vi "Vision Research Phantom Series PhCon Error Handler.vi"(0 "ErrNo":u32, 5 "Error In (no error)":errorcluster) -> (19 "Error Out":errorcluster)   [LabVIEW 2013, in "VRI.lvlib"]
doc: "This VI calls the PhGetErrorMessage function prototype for the PhCon.dll associated with the Vision Research Phantom Series cameras. An error message is created if an error code is returned.\n\nPlace this VI after any PhCon.dll call"
uses:
  VRI.lvlib
  Phantom DLLs/PhCon.Dll
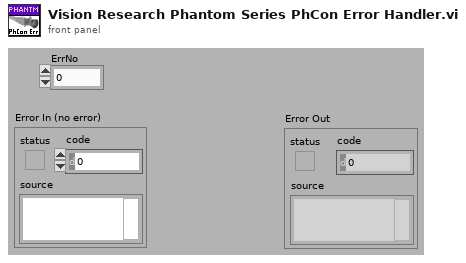
[diagram p1: front panel]
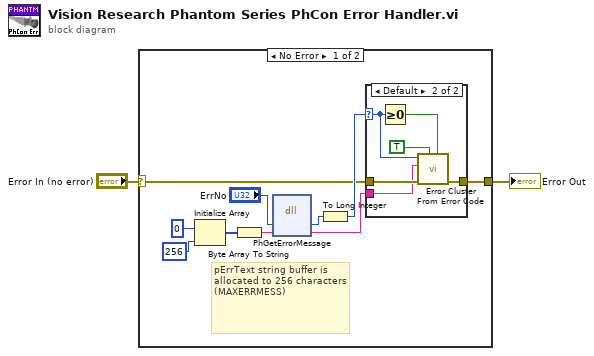
[diagram p0: block diagram]
diagram:
  n1 = case shown="No Error" "Error In (no error)" {
    selector: "Error In (no error)" -> [w3 w20]
    tunnel: [w12 w20] -> w2
    frame No Error {
      # "pErrText string buffer is allocated to 256 characters (MAXERRMESS)"
      n2 = Initialize Array(u8 0, 256 ("dimension size")) -> (w10:u8[])
      n3 = Byte Array To String(unsigned byte array=w10) -> (string=w7:string)
      n4 = dll-call lib="C:/Projects/SDK/64-bit/Vision Research Phantom Series Labview Driver/Phantom DLLs/PhCon.dll" fn="PhGetErrorMessage"("ErrNo"="ErrNo", "pErrText"=w7) -> ("ErrNo"=w9:u32, "pErrText"=w6:string)  [unwired: 3 in, 3 out]
      n5 = To Long Integer(number=w9) -> (32bit integer=w4:i32)
      n6 = case shown="Default" w4 {
        selector: w4 -> [_ w14]
        tunnel: w3 -> [w13 w19]
        tunnel: [w13 w18] -> w12
        tunnel: w6 -> [_ w17]
        frame 0 {
        }
        frame Default {
          n7 = Greater Or Equal To 0?(x=w14) -> (x >= 0?=w15:bool)
          n8 = call <vilib>:"Error Cluster From Error Code.vi"("is warning? (False)"=w15, "show call chain? (False)"=TRUE, "error in (no error)"=w19, "error message (\"\")"=w17, "error code (0)"=w14) -> ("error out"=w18:errorcluster)  [unwired: 4 in]
        }
      }
    }
    frame Error {
    }
  }
  "Error Out" <- w2
